vi "PrgSet.vi"(8 "error in (no error)":errorcluster, 9 "Tag":string, 10 "An Array of SEQ":refnum<class "Sequence.lvclass">[](array[class]), 11 "Program in":refnum<class "Program.lvclass">) -> (0 "error out":errorcluster, 3 "Program out":refnum<class "Program.lvclass">)   [LabVIEW 2012, in "Program.lvclass"]
uses:
  Program.lvclass
  Sequence.lvclass
  Program.lvclass/Program.ctl
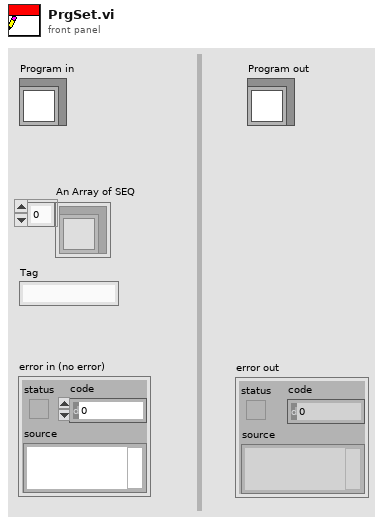
[diagram p1: front panel]
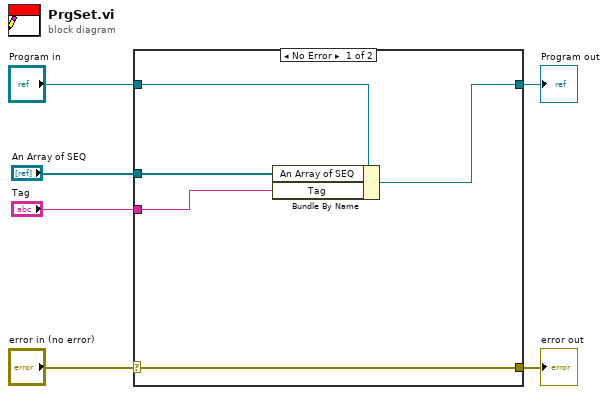
[diagram p0: block diagram]
diagram:
  n1 = case shown="No Error" "error in (no error)" {
    selector: "error in (no error)" -> [w11 w12]
    tunnel: [w11 w12] -> w5
    tunnel: [w9 w13] -> w3
    tunnel: "Program in" -> [w10 w13]
    tunnel: "An Array of SEQ" -> [w8 _]
    tunnel: "Tag" -> [w7 _]
    frame No Error {
      n2 = Bundle By Name(cluster=w10, "An Array of SEQ"=w8, "Tag"=w7) -> (w9:refnum<class "Program.lvclass">)
    }
    frame Error {
    }
  }
  "error out" <- w5
  "Program out" <- w3
